vi "Translater.vi"(1 "In":string, 2 "error in (no error)":errorcluster) -> (3 "Card":string, 5 "Comp":string, 6 "error out (no error)":errorcluster)   [LabVIEW 2011]
doc: "This vi are dividing the string to two separate strings one containing card number and the adder one contain components, and the vi are also translating the information to a format the circuit wiring robot can handle.\n\nExample: Connect component 2 & 5 on card 3 --> Circurit Builder --> following string: 3 18 \n--> Translater --> 003018000000"
uses:
  Server_Globals.vi
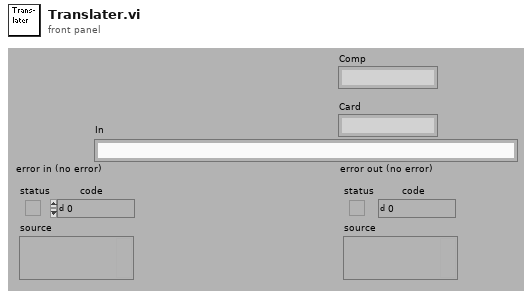
[diagram p1: front panel]
types:
  T1 = cluster{"I/O Settings":u64[], "Instrument Handle":cluster{"5402":refnum<k15>, " 5112":refnum<k15>, "4072":refnum<k15>, "USB":refnum<visa-resource-name>, "4110":refnum<k15>}, "Logfile":refnum<file>, "Log Level":i8, "Clear":i32[], "OS Set":cluster{"instrument handle out":refnum<k15>, "remaining string":string, "Settings":cluster{"Horizontal Conf.":cluster{"Min. Sample rate":dbl, "Reference position":dbl, "Record Length":i16}, "Channel A":cluster{"Enable":bool, "Vertical coupling":dbl, "Vertical range":dbl, "Vertical offset":dbl, "Probe attenuation":dbl}, "Channel B":cluster{"Enable":bool, "Vertical coupling":dbl, "Vertical range":dbl, "Vertical offset":dbl, "Probe attenuation":dbl}, "Trigger":cluster{"Source":enum8{"channel 1", "channel 2", "Imediate", "External trigger"}, "Slope":enum8{"Positive", "Negative"}, "Coupling":enum8{"AC", "DC"}, "Level":dbl, "Holdoff":dbl, "Delay":dbl, " Timeout":dbl, " Mode":enum8{"Normal", "Auto", "Auto Level"}}, "Measurements":cluster{"Measurement 1, Channel":enum8{"Channel 1", "Channel 2", "Channel 3", "Channel 4"}, "Measurement 1, Selection":u16, "Measurement 2, Channel":enum8{"Channel 1", "Channel 2", "Channel 3", "Channel 4"}, "Measurement 2,  Selection":u16, "Measurement 3, Channel":enum8{"Channel 1", "Channel 2", "Channel 3", "Channel 4"}, "Measurement 3, Selection 3":u16}}}, "DC Power Supply":cluster{"0":refnum<k15>, "1":refnum<k15>, "2":refnum<k15>, "3":refnum<k15>, "4":refnum<k15>}, "USB Interface":cluster{"0":refnum<visa-resource-name>, "1":refnum<visa-resource-name>, "2":refnum<visa-resource-name>, "3":refnum<visa-resource-name>, "4":refnum<visa-resource-name>}, "Function Generator":cluster{"0":refnum<k15>, "1":refnum<k15>, "2":refnum<k15>, "3":refnum<k15>, "4":refnum<k15>}, "Digital Multimeter":cluster{"0":refnum<k15>, "1":refnum<k15>, "2":refnum<k15>, "3":refnum<k15>, "4":refnum<k15>}, "Digital Osciliscope":cluster{"0":refnum<k15>, "1":refnum<k15>, "2":refnum<k15>, "3":refnum<k15>, "4":refnum<k15>}, "To M Server":string, "Adres":string[][], "Matrix version":string, "MD5":string, "Digital Multimeter Card 2":cluster{"0":string, "1":string, "2":string, "3":string, "4":string}}
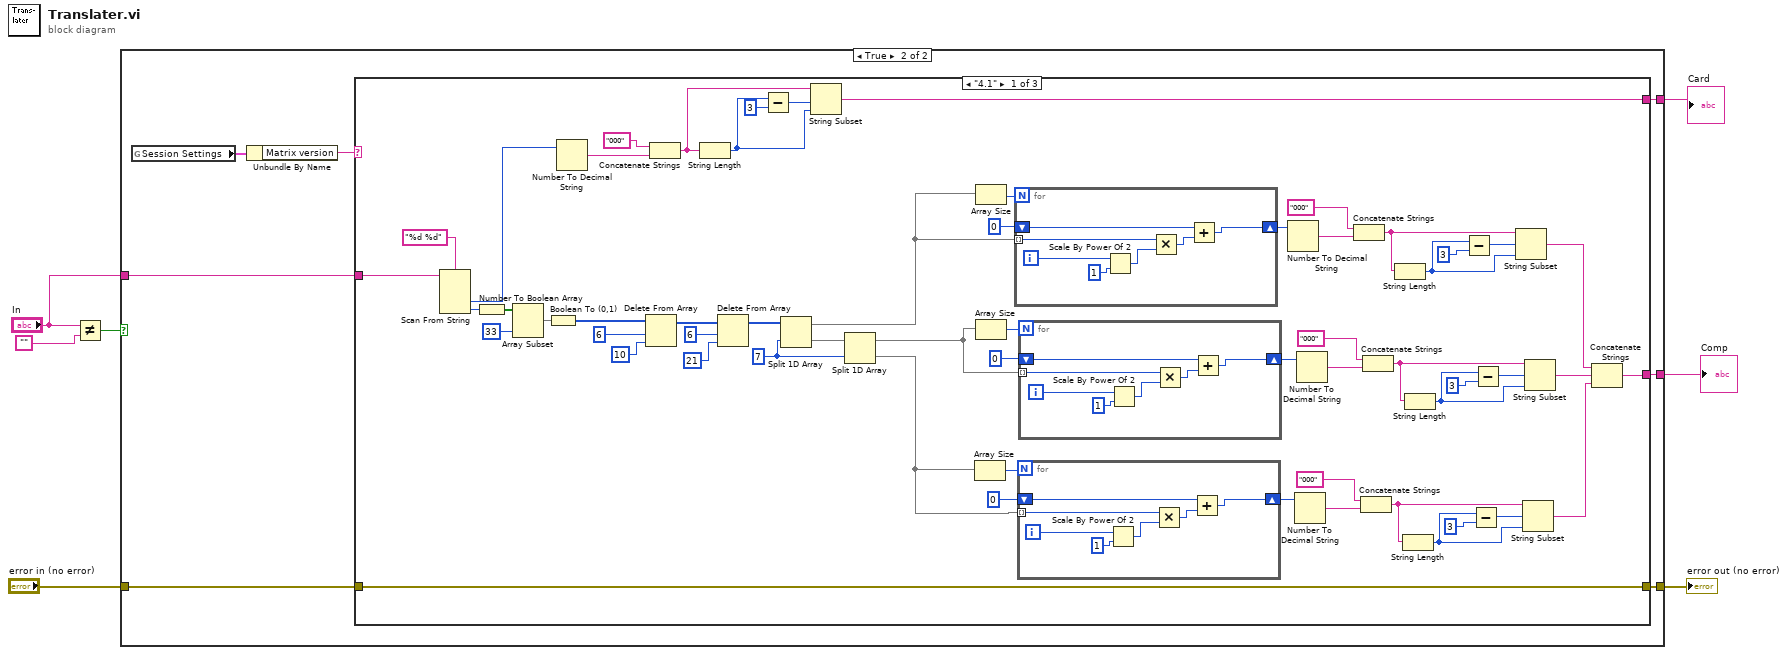
[diagram p0: block diagram]
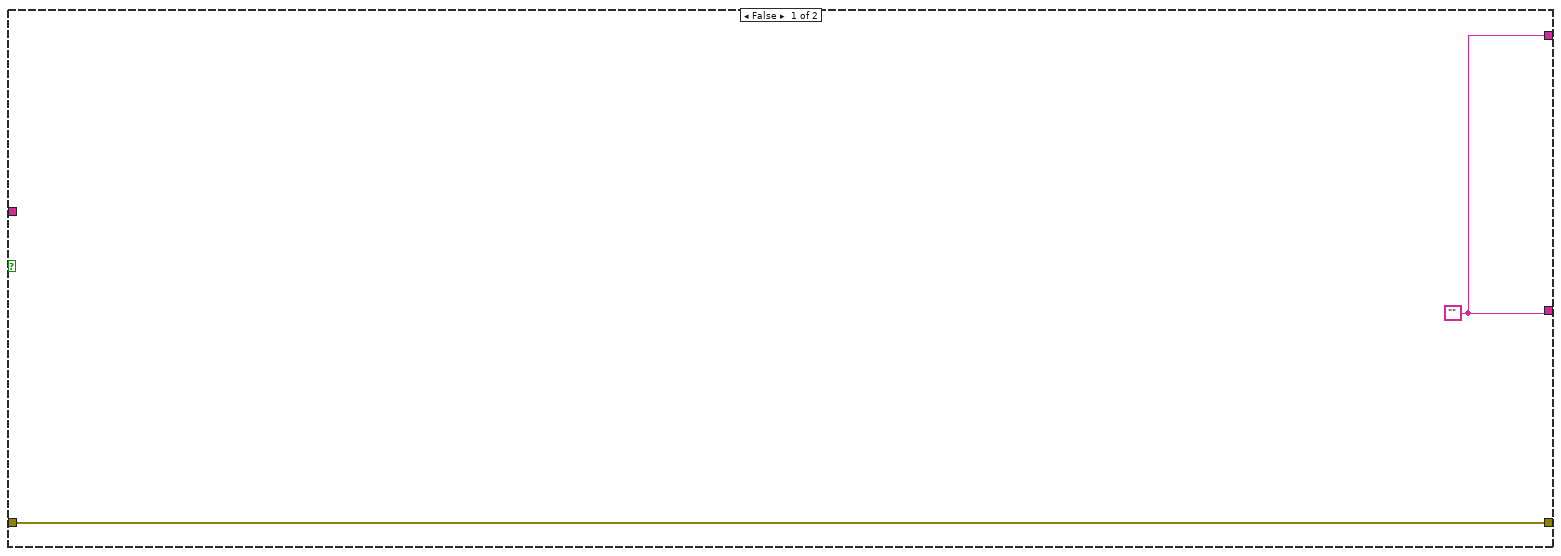
[diagram p2: hidden frame]
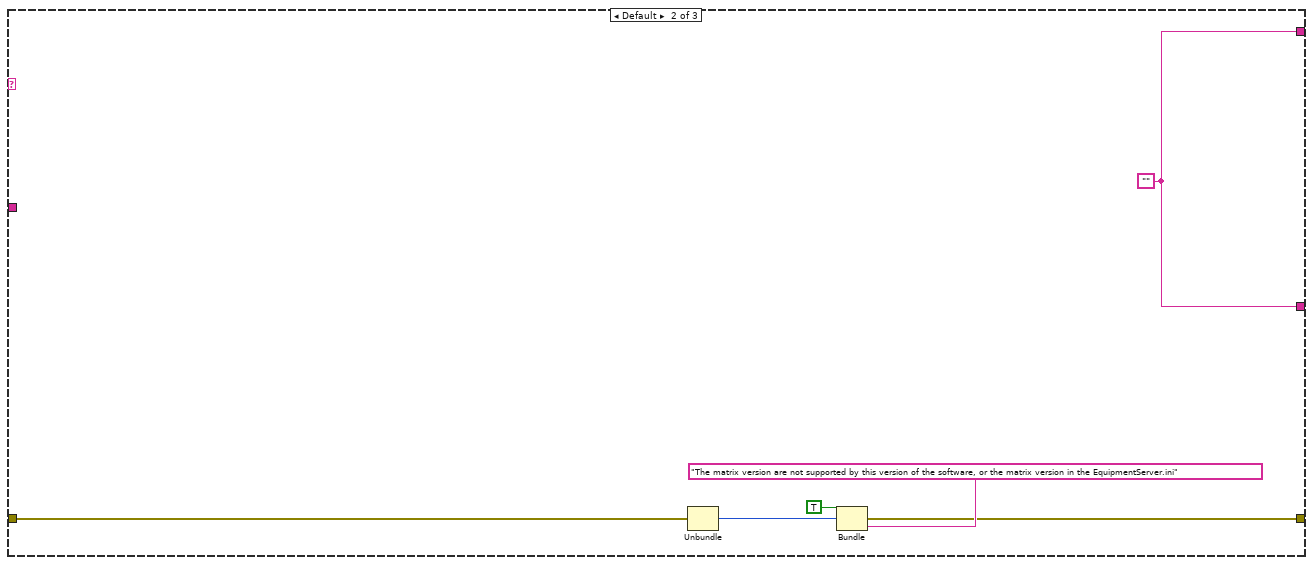
[diagram p3: hidden frame]
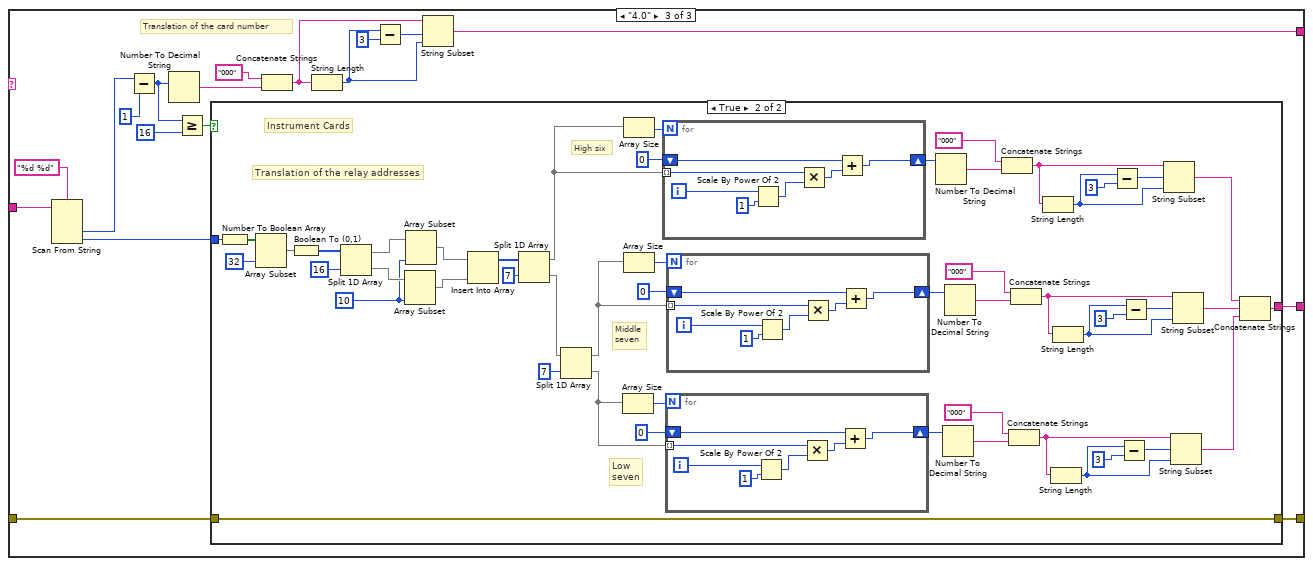
[diagram p4: hidden frame]
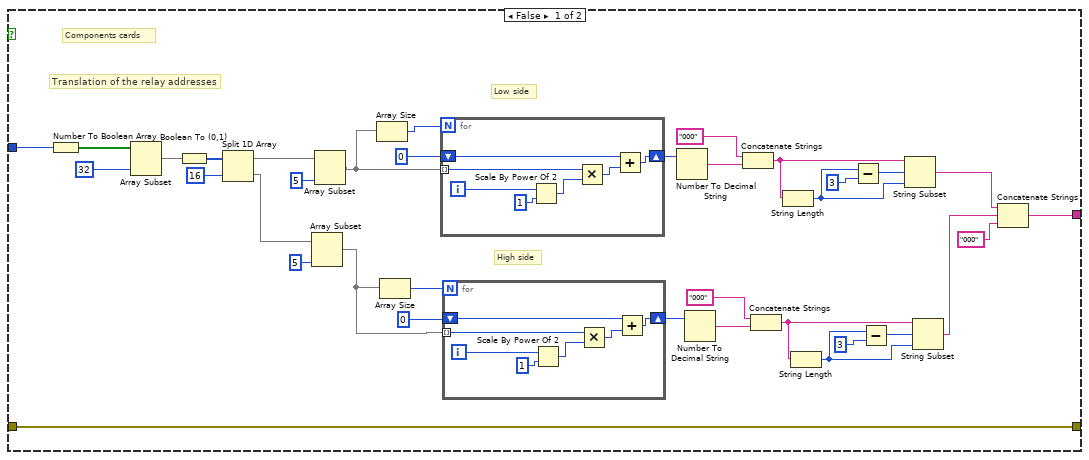
[diagram p5: hidden frame]
diagram:
  n1 = Not Equal?(x="In", y="") -> (x != y?=w5:bool)
  n2 = case shown="True" w5 {
    tunnel: [w9 w16] -> w7
    tunnel: [w9 w15] -> w6
    tunnel: "In" -> [_ w10]
    tunnel: "error in (no error)" -> [w8 w14]
    tunnel: [w8 w13] -> w1
    frame False {
      w9 = ""
    }
    frame True {
      n3 = global read "Server_Globals.vi" "Session Settings"() -> (w12:T1)
      n4 = Unbundle By Name(w12) -> ("Matrix version"=w11:string)
      n5 = case shown="\"4.1\"" w11 {
        tunnel: [w21 w96 w119] -> w16
        tunnel: [w65 w96 w108] -> w15
        tunnel: w10 -> [w66 _ w104]
        tunnel: w14 -> [w74 w97 w103]
        tunnel: [w74 w98 w102] -> w13
        frame "4.1" {
          w52 = 7
          n6 = Scan From String(format string="%d %d", input string=w66) -> (output 1=w17:i32, output 2=w61:i32)  [unwired: 4 in, 3 out]
          n7 = Number To Boolean Array(number=w61) -> (Boolean array=w64:bool[])
          n8 = Array Subset(array=w64, length=33) -> (w62:bool[])  [unwired: 1 in]
          n9 = Boolean To (0,1)(Boolean=w62) -> (0, 1=w60:i16[])
          n10 = Number To Decimal String(number=w17) -> (decimal integer string=w72:string)  [unwired: 1 in]
          n11 = Delete From Array(array=w60, length=6, index=10) -> (array with subset deleted=w57:i16[])  [unwired: 1 out]
          n12 = Concatenate Strings("000", w72) -> (w70:string)
          n13 = String Length(string=w70) -> (length=w67:i32)
          n14 = Delete From Array(array=w57, length=6, index=21) -> (array with subset deleted=w54:i16[])  [unwired: 1 out]
          n15 = Subtract(x=w67, y=3) -> (x-y=w69:i32)
          n16 = Split 1D Array(array=w54, index=w52) -> (first subarray=w20:i16[], second subarray=w53:i16[])
          n17 = String Subset(string=w70, offset (0)=w69, length (rest)=w67) -> (substring=w65:string)
          n18 = Split 1D Array(array=w53, index=w52) -> (first subarray=w19:i16[], second subarray=w18:i16[])
          n19 = Array Size(array=w18) -> (size(s)=w32:i32)
          n20 = Array Size(array=w20) -> (size(s)=w51:i32)
          n21 = Array Size(array=w19) -> (size(s)=w48:i32)
          n22 = for {
            N: w51 -> [_]
            shift-right: [w89] -> w50
            shift-left: 0 -> [w90]
            tunnel: w20 -> [w92] mode=indexing
            i -> [w95]
            n23 = Scale By Power Of 2(n=w95, x=1) -> (x*2^n=w93:i32)
            n24 = Multiply(x=w92, y=w93) -> (x*y=w91:i32)
            n25 = Add(x=w90, y=w91) -> (x+y=w89:i32)
          }
          n26 = for {
            N: w32 -> [_]
            shift-right: [w75] -> w25
            shift-left: 0 -> [w76]
            tunnel: w18 -> [w78] mode=indexing
            i -> [w81]
            n27 = Scale By Power Of 2(n=w81, x=1) -> (x*2^n=w79:i32)
            n28 = Multiply(x=w78, y=w79) -> (x*y=w77:i32)
            n29 = Add(x=w76, y=w77) -> (x+y=w75:i32)
          }
          n30 = for {
            N: w48 -> [_]
            shift-right: [w82] -> w34
            shift-left: 0 -> [w83]
            tunnel: w19 -> [w85] mode=indexing
            i -> [w88]
            n31 = Scale By Power Of 2(n=w88, x=1) -> (x*2^n=w86:i32)
            n32 = Multiply(x=w85, y=w86) -> (x*y=w84:i32)
            n33 = Add(x=w83, y=w84) -> (x+y=w82:i32)
          }
          n34 = Number To Decimal String(number=w50) -> (decimal integer string=w46:string)  [unwired: 1 in]
          n35 = Number To Decimal String(number=w25) -> (decimal integer string=w30:string)  [unwired: 1 in]
          n36 = Number To Decimal String(number=w34) -> (decimal integer string=w40:string)  [unwired: 1 in]
          n37 = Concatenate Strings("000", w46) -> (w44:string)
          n38 = Concatenate Strings("000", w30) -> (w29:string)
          n39 = Concatenate Strings("000", w40) -> (w38:string)
          n40 = String Length(string=w44) -> (length=w41:i32)
          n41 = String Length(string=w29) -> (length=w26:i32)
          n42 = String Length(string=w38) -> (length=w35:i32)
          n43 = Subtract(x=w41, y=3) -> (x-y=w43:i32)
          n44 = Subtract(x=w26, y=3) -> (x-y=w28:i32)
          n45 = Subtract(x=w35, y=3) -> (x-y=w37:i32)
          n46 = String Subset(string=w44, offset (0)=w43, length (rest)=w41) -> (substring=w22:string)
          n47 = String Subset(string=w29, offset (0)=w28, length (rest)=w26) -> (substring=w23:string)
          n48 = String Subset(string=w38, offset (0)=w37, length (rest)=w35) -> (substring=w33:string)
          n49 = Concatenate Strings(w22, w33, w23) -> (w21:string)
        }
        frame Default {
          w96 = ""
          n50 = Unbundle(w97) -> ("code"=w99:i32)  [unwired: 2 out]
          n51 = Bundle("status"=TRUE, "code"=w99, "The matrix version are not supported by this version of the software, or the matrix version in the EquipmentServer.ini") -> (w98:cluster{"status":bool, "code":i32, string})  [unwired: 1 in]
        }
        frame "4.0" {
          # "Translation of the card number"
          n52 = Scan From String(format string="%d %d", input string=w104) -> (output 1=w116:i32, output 2=w117:i32)  [unwired: 4 in, 3 out]
          n53 = Subtract(x=w116, y=1) -> (x-y=w106:i32)
          n54 = Number To Decimal String(number=w106) -> (decimal integer string=w114:string)  [unwired: 1 in]
          n55 = Greater Or Equal?(x=w106, y=16) -> (x >= y?=w107:bool)
          n56 = case shown="True" w107 {
            tunnel: [w131 w195] -> w119
            tunnel: w117 -> [w130 w181]
            tunnel: w103 -> [w120 w169]
            tunnel: [w120 w169] -> w102
            frame False {
              # "High side"
              # "Low side"
              # "Translation of the relay addresses"
              # "Components cards"
              n57 = Number To Boolean Array(number=w130) -> (Boolean array=w154:bool[])
              n58 = Array Subset(array=w154, length=32) -> (w152:bool[])  [unwired: 1 in]
              n59 = Boolean To (0,1)(Boolean=w152) -> (0, 1=w151:i16[])
              n60 = Split 1D Array(array=w151, index=16) -> (first subarray=w129:i16[], second subarray=w127:i16[])
              n61 = Array Subset(array=w127, length=5) -> (w126:i16[])  [unwired: 1 in]
              n62 = Array Subset(array=w129, length=5) -> (w128:i16[])  [unwired: 1 in]
              n63 = Array Size(array=w128) -> (size(s)=w149:i32)
              n64 = Array Size(array=w126) -> (size(s)=w146:i32)
              n65 = for {
                N: w149 -> [_]
                shift-right: [w162] -> w148
                shift-left: 0 -> [w163]
                tunnel: w128 -> [w165] mode=indexing
                i -> [w168]
                n66 = Scale By Power Of 2(n=w168, x=1) -> (x*2^n=w166:i32)
                n67 = Multiply(x=w165, y=w166) -> (x*y=w164:i32)
                n68 = Add(x=w163, y=w164) -> (x+y=w162:i32)
              }
              n69 = for {
                N: w146 -> [_]
                shift-right: [w155] -> w132
                shift-left: 0 -> [w156]
                tunnel: w126 -> [w158] mode=indexing
                i -> [w161]
                n70 = Scale By Power Of 2(n=w161, x=1) -> (x*2^n=w159:i32)
                n71 = Multiply(x=w158, y=w159) -> (x*y=w157:i32)
                n72 = Add(x=w156, y=w157) -> (x+y=w155:i32)
              }
              n73 = Number To Decimal String(number=w148) -> (decimal integer string=w144:string)  [unwired: 1 in]
              n74 = Number To Decimal String(number=w132) -> (decimal integer string=w138:string)  [unwired: 1 in]
              n75 = Concatenate Strings("000", w144) -> (w142:string)
              n76 = Concatenate Strings("000", w138) -> (w136:string)
              n77 = String Length(string=w142) -> (length=w139:i32)
              n78 = String Length(string=w136) -> (length=w133:i32)
              n79 = Subtract(x=w139, y=3) -> (x-y=w141:i32)
              n80 = Subtract(x=w133, y=3) -> (x-y=w135:i32)
              n81 = String Subset(string=w142, offset (0)=w141, length (rest)=w139) -> (substring=w123:string)
              n82 = String Subset(string=w136, offset (0)=w135, length (rest)=w133) -> (substring=w122:string)
              n83 = Concatenate Strings(w123, w122, "000") -> (w131:string)
            }
            frame True {
              w176 = 10
              # "Low\nseven"
              # "Middle\nseven"
              # "High six"
              # "Translation of the relay addresses"
              # "Instrument Cards"
              n84 = Number To Boolean Array(number=w181) -> (Boolean array=w218:bool[])
              n85 = Array Subset(array=w218, length=32) -> (w216:bool[])  [unwired: 1 in]
              n86 = Boolean To (0,1)(Boolean=w216) -> (0, 1=w180:i16[])
              n87 = Split 1D Array(array=w180, index=16) -> (first subarray=w178:i16[], second subarray=w177:i16[])
              n88 = Array Subset(array=w177, length=w176) -> (w173:i16[])  [unwired: 1 in]
              n89 = Array Subset(array=w178, length=w176) -> (w174:i16[])  [unwired: 1 in]
              n90 = Insert Into Array(array=w174, new element=w173) -> (w175:i16[])  [unwired: 1 in]
              n91 = Split 1D Array(array=w175, index=7) -> (first subarray=w214:i16[], second subarray=w194:i16[])
              n92 = Split 1D Array(array=w194, index=7) -> (first subarray=w192:i16[], second subarray=w182:i16[])
              n93 = Array Size(array=w182) -> (size(s)=w191:i32)
              n94 = Array Size(array=w214) -> (size(s)=w215:i32)
              n95 = Array Size(array=w192) -> (size(s)=w211:i32)
              n96 = for {
                N: w215 -> [_]
                shift-right: [w233] -> w213
                shift-left: 0 -> [w234]
                tunnel: w214 -> [w236] mode=indexing
                i -> [w239]
                n97 = Scale By Power Of 2(n=w239, x=1) -> (x*2^n=w237:i32)
                n98 = Multiply(x=w236, y=w237) -> (x*y=w235:i32)
                n99 = Add(x=w234, y=w235) -> (x+y=w233:i32)
              }
              n100 = for {
                N: w191 -> [_]
                shift-right: [w219] -> w184
                shift-left: 0 -> [w220]
                tunnel: w182 -> [w222] mode=indexing
                i -> [w225]
                n101 = Scale By Power Of 2(n=w225, x=1) -> (x*2^n=w223:i32)
                n102 = Multiply(x=w222, y=w223) -> (x*y=w221:i32)
                n103 = Add(x=w220, y=w221) -> (x+y=w219:i32)
              }
              n104 = for {
                N: w211 -> [_]
                shift-right: [w226] -> w197
                shift-left: 0 -> [w227]
                tunnel: w192 -> [w229] mode=indexing
                i -> [w232]
                n105 = Scale By Power Of 2(n=w232, x=1) -> (x*2^n=w230:i32)
                n106 = Multiply(x=w229, y=w230) -> (x*y=w228:i32)
                n107 = Add(x=w227, y=w228) -> (x+y=w226:i32)
              }
              n108 = Number To Decimal String(number=w213) -> (decimal integer string=w209:string)  [unwired: 1 in]
              n109 = Number To Decimal String(number=w184) -> (decimal integer string=w189:string)  [unwired: 1 in]
              n110 = Number To Decimal String(number=w197) -> (decimal integer string=w203:string)  [unwired: 1 in]
              n111 = Concatenate Strings("000", w209) -> (w207:string)
              n112 = Concatenate Strings("000", w189) -> (w188:string)
              n113 = Concatenate Strings("000", w203) -> (w201:string)
              n114 = String Length(string=w207) -> (length=w204:i32)
              n115 = String Length(string=w188) -> (length=w185:i32)
              n116 = String Length(string=w201) -> (length=w198:i32)
              n117 = Subtract(x=w204, y=3) -> (x-y=w206:i32)
              n118 = Subtract(x=w185, y=3) -> (x-y=w187:i32)
              n119 = Subtract(x=w198, y=3) -> (x-y=w200:i32)
              n120 = String Subset(string=w207, offset (0)=w206, length (rest)=w204) -> (substring=w170:string)
              n121 = String Subset(string=w188, offset (0)=w187, length (rest)=w185) -> (substring=w171:string)
              n122 = String Subset(string=w201, offset (0)=w200, length (rest)=w198) -> (substring=w196:string)
              n123 = Concatenate Strings(w170, w196, w171) -> (w195:string)
            }
          }
          n124 = Concatenate Strings("000", w114) -> (w112:string)
          n125 = String Length(string=w112) -> (length=w109:i32)
          n126 = Subtract(x=w109, y=3) -> (x-y=w111:i32)
          n127 = String Subset(string=w112, offset (0)=w111, length (rest)=w109) -> (substring=w108:string)
        }
      }
    }
  }
  "Comp" <- w7
  "Card" <- w6
  "error out (no error)" <- w1
